vi "Teleop.vi"(10 "Match Info":T1={"Autonomous Elapsed Seconds"=0.0, "TeleOp Elapsed Seconds"=0.0, "Disabled Elapsed Seconds"=0.0, "Visited Autonomous"=FALSE, "Visited TeleOp"=FALSE, "Visited Disabled"=FALSE, "Autonomous Settings"={"Autonomous Style"=enum."Independent", "VI Refnum"=refnum}}, 11 "Call Context":T2) -> ()   [LabVIEW 2020]
doc: "This VI is called for each TeleOp packet received from the DS where the robot is not disabled. It is often used to read from the joysticks and update I/O or to update setpoints for timed control loops. It should complete and return within 20 milliseconds or it may miss DS packets."
uses:
  <vilib>/Rock Robotics/WPI/DriverStation/WPI_DriverStationDerivedRobotMode.ctl
  <vilib>/Rock Robotics/WPI/DriverStation/WPI_DriverStationMatch Info.ctl
  Robot Global Data.vi
panel:
  out "Numeric":dbl
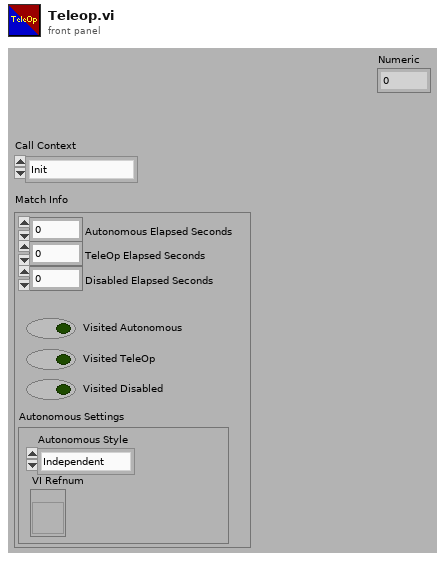
[diagram p1: front panel]
types:
  T1 = typedef "WPI_DriverStationMatch Info.ctl" = cluster{"Autonomous Elapsed Seconds":dbl, "TeleOp Elapsed Seconds":dbl, "Disabled Elapsed Seconds":dbl, "Visited Autonomous":bool, "Visited TeleOp":bool, "Visited Disabled":bool, "Autonomous Settings":cluster{"Autonomous Style":enum16{"Iterative", "Independent"}, "VI Refnum":refnum<vi>}}
  T2 = typedef "WPI_DriverStationDerivedRobotMode.ctl" = enum16{"Init", "Execute", "Stop"}
  T3 = typedef "WPI_ServoDeviceRef.ctl" = cluster{"DeviceStatus":errorcluster, "PWM Channel":T4, "DeadBand":T5}
  T4 = typedef "FPGA_DIOPWMChannel.ctl" = enum8{"PWM 0", "PWM 1", "PWM 2", "PWM 3", "PWM 4", "PWM 5", "PWM 6", "PWM 7", "PWM 8", "PWM 9", "PWM MXP 0", "PWM MXP 1", "PWM MXP 2", "PWM MXP 3", "PWM MXP 4", "PWM MXP 5", "PWM MXP 6", "PWM MXP 7", "PWM MXP 8", "PWM MXP 9", "Invalid"}
  T5 = typedef "WPI_PWMDeadband.ctl" = cluster{"Name":string, "maxPositivePwm":i32, "minPositivePwm":i32, "centerPwm":i32, "maxNegativePwm":i32, "minNegativePwm":i32, "angularRange":u16}
  T6 = typedef "WPI_JoystickDevRef.ctl" = cluster{"Device":T7}
  T7 = typedef "WPI_JoystickDeviceEnum.ctl" = enum16{"USB 0", "USB 1", "USB 2", "USB 3", "USB 4", "USB 5"}
  T8 = typedef "WPI_MotorControlDeviceRef.ctl" = cluster{"DeviceStatus":errorcluster, "Type":T9, "PWM":cluster{"PWM Channel":T4, "DeadBand":T5}, "CAN":cluster{"Device Number":u8, "SetOutput VI Ref":variant, "GetOutput VI Ref":variant, "Enable VI Ref":variant, "Disable VI Ref":variant, "Data":variant}, "Invert":bool, "DIO PWM":cluster{"PWM \"Enable\" Channel":T4, "DIOChannel":T10, "PWM Rate":dbl}}
  T9 = typedef "WPI_MotorControlType.ctl" = enum16{"PWM", "CAN", "DIO PWM"}
  T10 = typedef "FPGA_DIOChannel.ctl" = enum8{"DIO 0", "DIO 1", "DIO 2", "DIO 3", "DIO 4", "DIO 5", "DIO 6", "DIO 7", "DIO 8", "DIO 9", "DIO MXP 0", "DIO MXP 1", "DIO MXP 2", "DIO MXP 3", "DIO MXP 4", "DIO MXP 5", "DIO MXP 6", "DIO MXP 7", "DIO MXP 8", "DIO MXP 9", "DIO MXP 10", "DIO MXP 11", "DIO MXP 12", "DIO MXP 13", "DIO MXP 14", "DIO MXP 15", "SPI Port CS1", "SPI Port CS2", "SPI Port CS3", "SPI Port MISO", "SPI Port MOSI", "Invalid"}
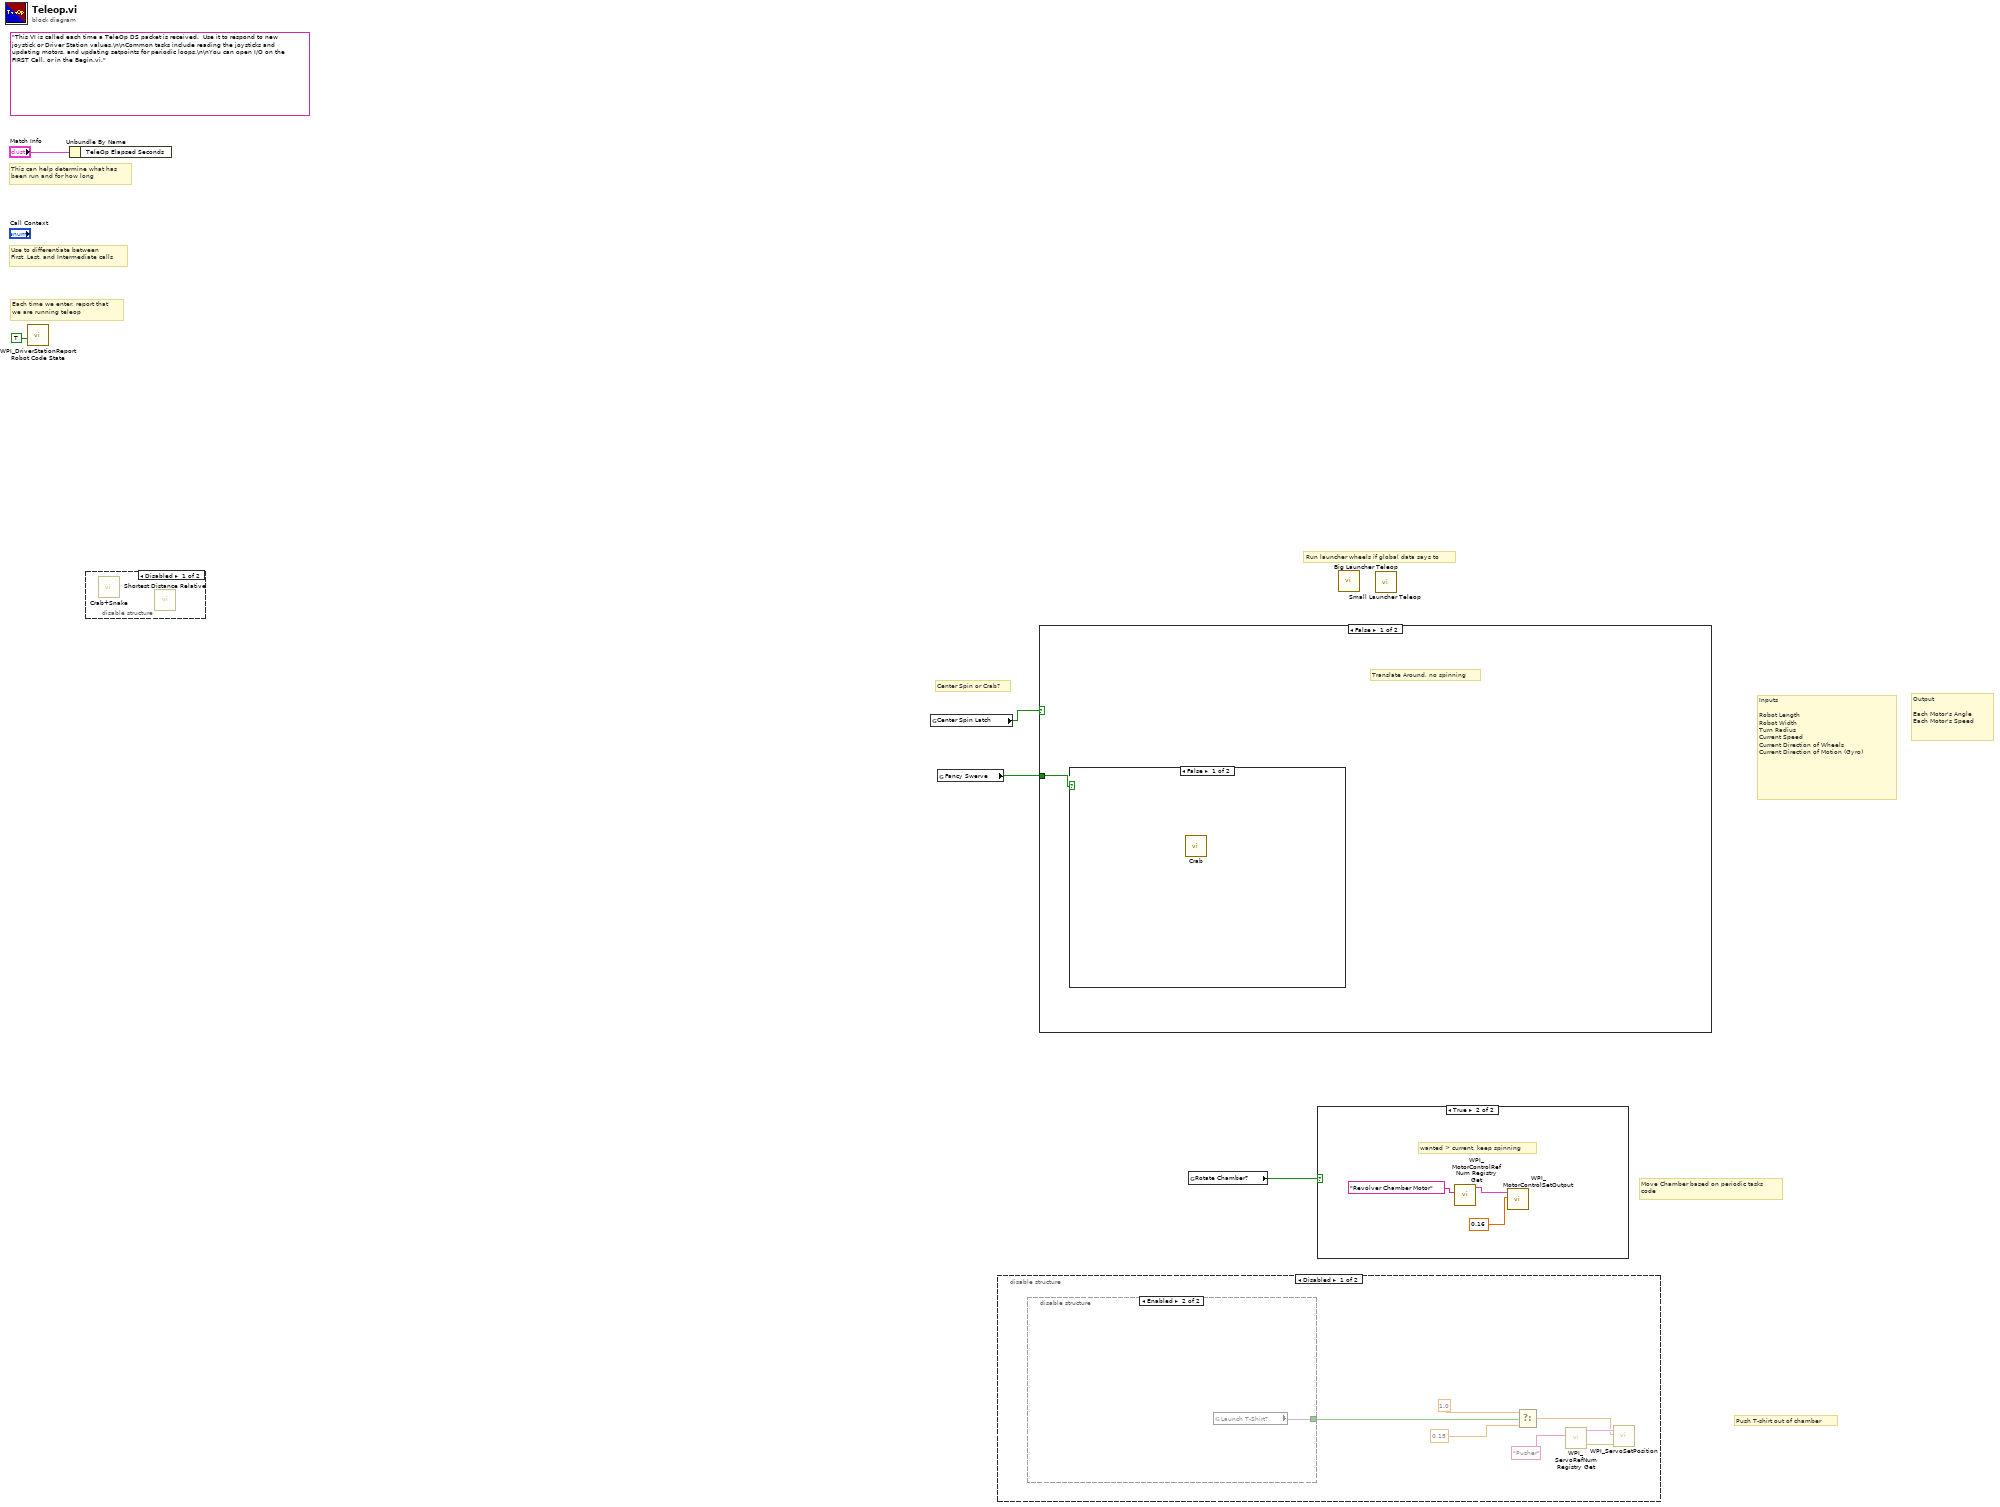
[diagram p0: block diagram]
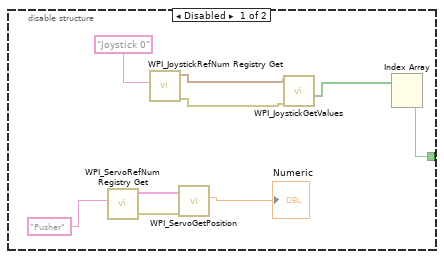
[diagram p2: hidden frame]
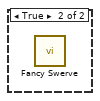
[diagram p4: hidden frame]
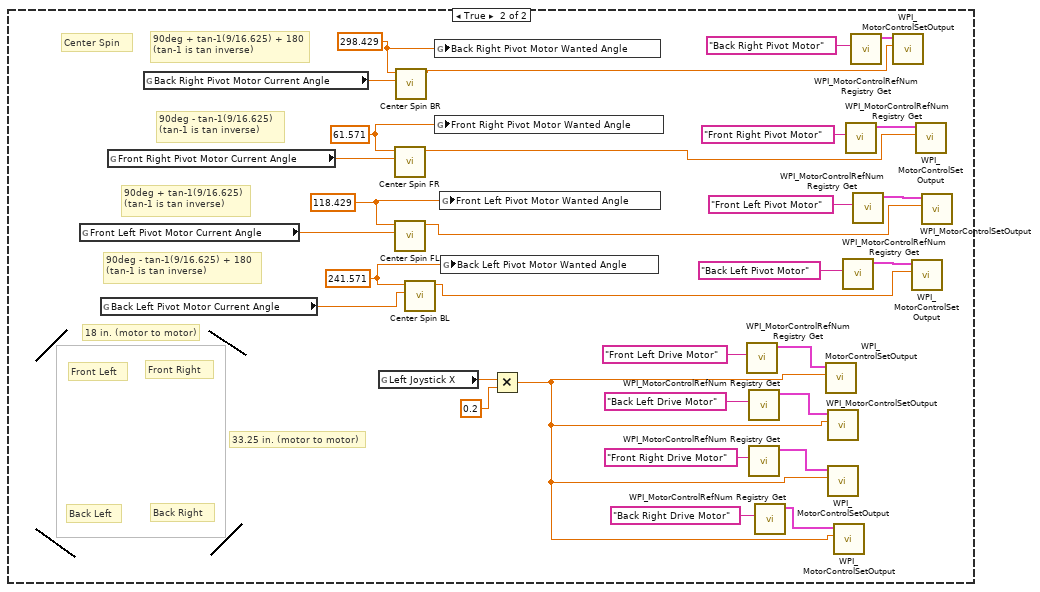
[diagram p5: hidden frame]
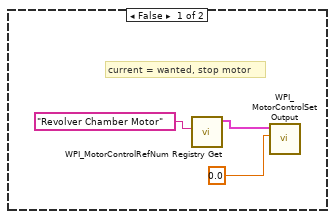
[diagram p6: hidden frame]
diagram:
  (unwired) "This VI is called each time a TeleOp DS packet is received.  Use it to respond to new joystick or Driver Station values.\n\nCommon tasks include reading the joysticks and updating motors, and updating setpoints for periodic loops.\n\nYou can open I/O on the FIRST Call, or in the Begin.vi."
  # "Output\n\nEach Motor's Angle\nEach Motor's Speed"
  # "Inputs\n\nRobot Length\nRobot Width\nTurn Radius\nCurrent Speed\nCurrent Direction of Wheels\nCurrent Direction of Motion (Gyro)"
  # "Push T-shirt out of chamber"
  # "Center Spin or Crab?"
  # "Run launcher wheels if global data says to"
  # "Move Chamber based on periodic tasks\ncode"
  # "Each time we enter, report that\nwe are running teleop"
  # "Use to differentiate between\nFirst, Last, and Intermediate calls"
  # "This can help determine what has\nbeen run and for how long"
  n1 = call <vilib>:"WPI_DriverStationReport Robot Code State.vi"("TeleOp"=TRUE ("Autonomous")) -> ()  [unwired: 10 in, 1 out]
  n2 = Unbundle By Name("Match Info") -> ()  [unwired: 1 out]
  n3 = disable-structure shown="Disabled" {
    frame Disabled {
      n4 = call "Crab+Snake.vi"() -> ()  [unwired: 10 in, 10 out]
      n5 = call "Shortest Distance Relative.vi"() -> ()  [unwired: 2 in, 10 out]
    }
    frame Enabled {
    }
  }
  n6 = global read "Robot Global Data.vi" "Center Spin Latch"() -> (w2:bool)
  n7 = global read "Robot Global Data.vi" "Fancy Swerve"() -> (w1:bool)
  n8 = disable-structure shown="Disabled" {
    frame Disabled {
      n9 = disable-structure shown="Enabled" {
        disable-tunnel: [w17 w22] -> w6
        frame Disabled {
          n10 = call <vilib>:"WPI_ServoRefNum Registry Get.vi"("refnum name"="Pusher") -> ("error out"=w16:errorcluster, "ServoDeviceRef"=w14:T3)  [unwired: 9 in]
          n11 = call <vilib>:"WPI_JoystickRefNum Registry Get.vi"("refnum name"="Joystick 0") -> ("error out"=w19:errorcluster, "JoystickDevRef"=w20:T6)  [unwired: 9 in]
          n12 = call <vilib>:"WPI_ServoGetPosition.vi"("error in (no error)"=w16, "ServoDeviceRef"=w14) -> ("Position"=→"Numeric":dbl)  [unwired: 7 in, 2 out]
          n13 = call <vilib>:"WPI_JoystickGetValues.vi"("error in (no error)"=w19, "JoystickDevRef"=w20) -> ("Buttons"=w18:bool[])  [unwired: 5 in, 4 out]
          n14 = Index Array(array=w18) -> (element #2=w17:bool)  [unwired: 2 in, 1 out]
        }
        frame Enabled {
          n15 = global read "Robot Global Data.vi" "Launch T-Shirt?"() -> (w22)
        }
      }
      n16 = Select(t=1.0 ("Extend Servo"), s=w6, f=0.15 ("Retract Servo")) -> (s? t:f=w8:dbl)
      n17 = call <vilib>:"WPI_ServoRefNum Registry Get.vi"("refnum name"="Pusher") -> ("error out"=w7:errorcluster, "ServoDeviceRef"=w9:T3)  [unwired: 9 in]
      n18 = call <vilib>:"WPI_ServoSetPosition.vi"("error in (no error)"=w7, "Position"=w8, "ServoDeviceRef"=w9) -> ()  [unwired: 7 in, 2 out]
    }
    frame Enabled {
    }
  }
  n19 = case shown="False" w2 {
    tunnel: w1 -> [w23 _]
    frame False {
      # "Translate Around, no spinning"
      n20 = case shown="False" w23 {
        frame False {
          n21 = call "Crab.vi"() -> ()  [unwired: 12 in]
        }
        frame True {
          n22 = call "Fancy Swerve.vi"() -> ()  [unwired: 12 in]
        }
      }
    }
    frame True {
      w27 = 241.571
      w26 = 118.429
      w25 = 61.571
      w24 = 298.429
      # "90deg - tan-1(9/16.625) + 180\n(tan-1 is tan inverse)"
      # "90deg + tan-1(9/16.625) + 180\n(tan-1 is tan inverse)"
      # "90deg - tan-1(9/16.625)\n(tan-1 is tan inverse)"
      # "33.25 in. (motor to motor)"
      # "18 in. (motor to motor)"
      # "90deg + tan-1(9/16.625)\n(tan-1 is tan inverse)"
      # "Center Spin"
      # "Back Right"
      # "Back Left"
      # "Front Right"
      # "Front Left"
      n23 = global read "Robot Global Data.vi" "Front Left Pivot Motor Current Angle"() -> (w37:dbl)
      n24 = global read "Robot Global Data.vi" "Back Left Pivot Motor Current Angle"() -> (w29:dbl)
      n25 = global read "Robot Global Data.vi" "Front Right Pivot Motor Current Angle"() -> (w38:dbl)
      n26 = global read "Robot Global Data.vi" "Back Right Pivot Motor Current Angle"() -> (w39:dbl)
      n27 = global read "Robot Global Data.vi" "Left Joystick X"() -> (w36:dbl)
      n28 = call "Center Spin FR.vi"("Wanted Angle"=w25, "Current Angle"=w38) -> ("Motor Output"=w41:dbl)  [unwired: 8 in]
      n29 = call "Center Spin FL.vi"("Wanted Angle"=w26, "Current Angle"=w37) -> ("Motor Output"=w40:dbl)  [unwired: 8 in]
      n30 = call "Center Spin BR.vi"("Wanted Angle"=w24, "Current Angle"=w39) -> ("Motor Output"=w42:dbl)  [unwired: 8 in]
      n31 = call "Center Spin BL.vi"("Wanted Angle"=w27, "Current Angle"=w29) -> ("Motor Output"=w28:dbl)  [unwired: 8 in]
      n32 = global write "Robot Global Data.vi" "Back Right Pivot Motor Wanted Angle"(w24) -> ()
      n33 = global write "Robot Global Data.vi" "Front Right Pivot Motor Wanted Angle"(w25) -> ()
      n34 = global write "Robot Global Data.vi" "Front Left Pivot Motor Wanted Angle"(w26) -> ()
      n35 = global write "Robot Global Data.vi" "Back Left Pivot Motor Wanted Angle"(w27) -> ()
      n36 = Multiply(x=w36, y=0.2) -> (x*y=w33:dbl)
      n37 = call <vilib>:"WPI_MotorControlRefNum Registry Get.vi"("refnum name"="Front Left Drive Motor") -> ("MotorControlDevRef"=w47:T8)  [unwired: 9 in, 1 out]
      n38 = call <vilib>:"WPI_MotorControlRefNum Registry Get.vi"("refnum name"="Back Left Drive Motor") -> ("MotorControlDevRef"=w51:T8)  [unwired: 9 in, 1 out]
      n39 = call <vilib>:"WPI_MotorControlRefNum Registry Get.vi"("refnum name"="Front Right Drive Motor") -> ("MotorControlDevRef"=w43:T8)  [unwired: 9 in, 1 out]
      n40 = call <vilib>:"WPI_MotorControlRefNum Registry Get.vi"("refnum name"="Back Right Drive Motor") -> ("MotorControlDevRef"=w30:T8)  [unwired: 9 in, 1 out]
      n41 = call <vilib>:"WPI_MotorControlSetOutput.vi"("Output"=w33, "MotorControlDevRef"=w47) -> ()  [unwired: 7 in, 3 out]
      n42 = call <vilib>:"WPI_MotorControlSetOutput.vi"("Output"=w33, "MotorControlDevRef"=w51) -> ()  [unwired: 7 in, 3 out]
      n43 = call <vilib>:"WPI_MotorControlSetOutput.vi"("Output"=w33, "MotorControlDevRef"=w43) -> ()  [unwired: 7 in, 3 out]
      n44 = call <vilib>:"WPI_MotorControlSetOutput.vi"("Output"=w33, "MotorControlDevRef"=w30) -> ()  [unwired: 7 in, 3 out]
      n45 = call <vilib>:"WPI_MotorControlRefNum Registry Get.vi"("refnum name"="Back Left Pivot Motor") -> ("MotorControlDevRef"=w31:T8)  [unwired: 9 in, 1 out]
      n46 = call <vilib>:"WPI_MotorControlRefNum Registry Get.vi"("refnum name"="Front Right Pivot Motor") -> ("MotorControlDevRef"=w45:T8)  [unwired: 9 in, 1 out]
      n47 = call <vilib>:"WPI_MotorControlRefNum Registry Get.vi"("refnum name"="Back Right Pivot Motor") -> ("MotorControlDevRef"=w53:T8)  [unwired: 9 in, 1 out]
      n48 = call <vilib>:"WPI_MotorControlRefNum Registry Get.vi"("refnum name"="Front Left Pivot Motor") -> ("MotorControlDevRef"=w49:T8)  [unwired: 9 in, 1 out]
      n49 = call <vilib>:"WPI_MotorControlSetOutput.vi"("Output"=w42, "MotorControlDevRef"=w53) -> ()  [unwired: 7 in, 3 out]
      n50 = call <vilib>:"WPI_MotorControlSetOutput.vi"("Output"=w28, "MotorControlDevRef"=w31) -> ()  [unwired: 7 in, 3 out]
      n51 = call <vilib>:"WPI_MotorControlSetOutput.vi"("Output"=w41, "MotorControlDevRef"=w45) -> ()  [unwired: 7 in, 3 out]
      n52 = call <vilib>:"WPI_MotorControlSetOutput.vi"("Output"=w40, "MotorControlDevRef"=w49) -> ()  [unwired: 7 in, 3 out]
    }
  }
  n53 = global read "Robot Global Data.vi" "Rotate Chamber?"() -> (w3:bool)
  n54 = case shown="True" w3 {
    frame False {
      # "current = wanted, stop motor"
      n55 = call <vilib>:"WPI_MotorControlRefNum Registry Get.vi"("refnum name"="Revolver Chamber Motor") -> ("MotorControlDevRef"=w56:T8)  [unwired: 9 in, 1 out]
      n56 = call <vilib>:"WPI_MotorControlSetOutput.vi"("Output"=0.0, "MotorControlDevRef"=w56) -> ()  [unwired: 7 in, 3 out]
    }
    frame True {
      # "wanted > current, keep spinning"
      n57 = call <vilib>:"WPI_MotorControlRefNum Registry Get.vi"("refnum name"="Revolver Chamber Motor") -> ("MotorControlDevRef"=w59:T8)  [unwired: 9 in, 1 out]
      n58 = call <vilib>:"WPI_MotorControlSetOutput.vi"("Output"=0.16, "MotorControlDevRef"=w59) -> ()  [unwired: 7 in, 3 out]
    }
  }
  n59 = call "Big Launcher Teleop.vi"() -> ()  [unwired: 12 in]
  n60 = call "Small Launcher Teleop.vi"() -> ()  [unwired: 12 in]
